vi "ArduinoLT_Collect_Control.vi"(7 "Arduino Configuration":T2={"Lights: Digital I/O Pins"={"Coaxial"=0, "Spotlights"=0}, "Thermistor Settings"={"Analogue Readout Pin"=1, "Vcc Reference Pin"=0, "Paired Resistance (10K Ohms)"=10000.0, "Units (C)"=enum."Celsius"}} {"Thermistor Settings"."Paired Resistance (10K Ohms)" format="%#_13g"}, 8 "error in":errorcluster, 9 "Arduino Resource IN":T3={"VISA resource"="", "Board Type"=enum."Uno", "Connection Type"=enum."USB / Serial", "Bytes Per Packet (15)"=15}, 10 "Spotlights":bool, 11 "Coaxial light":bool) -> (0 "error out":errorcluster, 1 "Arduino Resource OUT":T3={"VISA resource"="COM11", "Board Type"=enum."Uno", "Connection Type"=enum."USB / Serial", "Bytes Per Packet (15)"=15}, 3 "Thermometer [C]":dbl(slide) scale=0.0..50.0)   [LabVIEW 2016]
uses:
  <vilib>/LabVIEW Interface for Arduino/Type Defs/Arduino Resource.ctl
  <vilib>/LabVIEW Interface for Arduino/Type Defs/Board Type.ctl
  Controls/ArduinoLT-ConfigurationControl.ctl
  <vilib>/LabVIEW Interface for Arduino/LabVIEW Interface for Arduino.lvlib
panel:
  in  "Tab Control":T1(tab)
  out "VCC [V]":dbl=5.0 format="%#_13g"
  # "LIGHTS"
  # "TEMPERATURE"
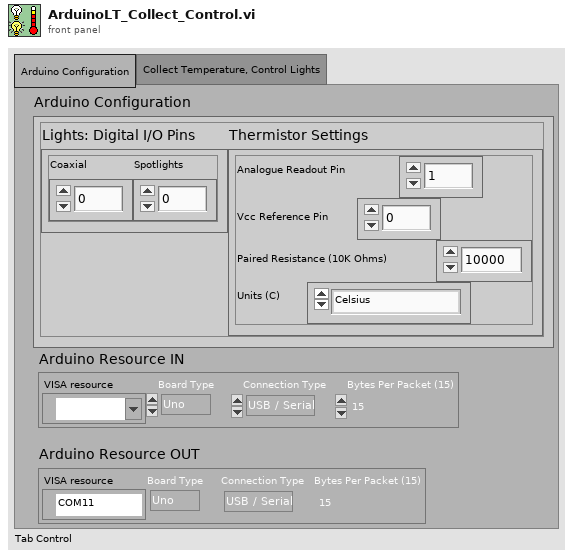
[diagram p1: front panel]
types:
  T1 = enum32{"Arduino Configuration", "Collect Temperature, Control Lights"}
  T2 = typedef "ArduinoLT-ConfigurationControl.ctl" = cluster{"Lights: Digital I/O Pins":cluster{"Coaxial":u8, "Spotlights":u8}, "Thermistor Settings":cluster{"Analogue Readout Pin":u8, "Vcc Reference Pin":u8, "Paired Resistance (10K Ohms)":dbl, "Units (C)":enum16{"Celsius", "Fahrenheit", "Kelvin"}}}
  T3 = typedef "LabVIEW Interface for Arduino.lvlib/Arduino Resource.ctl" = cluster{"VISA resource":refnum<visa-resource-name>, "Board Type":T4, "Connection Type":enum8{"USB / Serial"}, "Bytes Per Packet (15)":u8}
  T4 = typedef "LabVIEW Interface for Arduino.lvlib/Board Type.ctl" = enum16{"Uno", "Dimuelanove w/Atmega 328", "Mega 2560"}
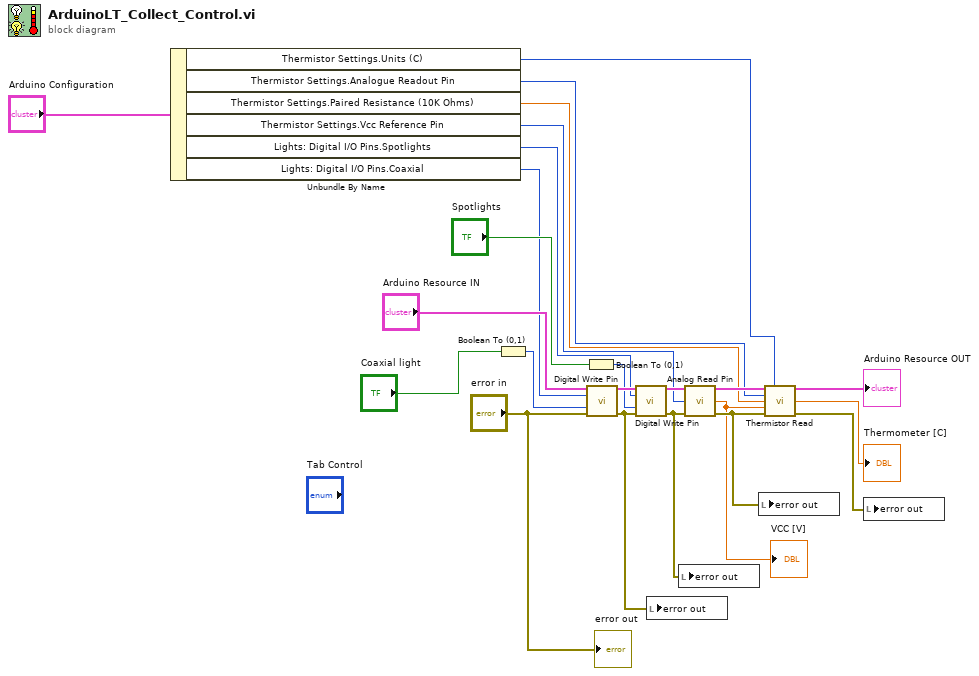
[diagram p0: block diagram]
diagram:
  n1 = Unbundle By Name("Arduino Configuration") -> ("Thermistor Settings.Units (C)"=w3:enum16{"Celsius", "Fahrenheit", "Kelvin"}, "Thermistor Settings.Analogue Readout Pin"=w4:u8, "Thermistor Settings.Paired Resistance (10K Ohms)"=w5:dbl, "Thermistor Settings.Vcc Reference Pin"=w6:u8, "Lights: Digital I/O Pins.Spotlights"=w7:u8, "Lights: Digital I/O Pins.Coaxial"=w8:u8)
  n2 = Boolean To (0,1)(Boolean="Coaxial light") -> (0, 1=w18:i16)
  n3 = Boolean To (0,1)(Boolean="Spotlights") -> (0, 1=w17:i16)
  n4 = call <vilib>:"Digital Write Pin.vi"("Arduino Resource"="Arduino Resource IN", "Digital I/O Pin (0)"=w8, "Value (0)"=w18, "error in"="error in") -> ("Arduino Resource"=w20:T3, "error out"=w11:errorcluster)  [unwired: 10 in]
  n5 = call <vilib>:"Digital Write Pin.vi"("Arduino Resource"=w20, "Digital I/O Pin (0)"=w7, "Value (0)"=w17, "error in"=w11) -> ("Arduino Resource"=w16:T3, "error out"=w12:errorcluster)  [unwired: 10 in]
  n6 = local write "error out"(w11) -> ()
  n7 = local write "error out"(w12) -> ()
  n8 = call <vilib>:"Analog Read Pin.vi"("Arduino Resource"=w16, "Analog Input Pin (0)"=w6, "error in"=w12) -> ("Arduino Resource"=w15:T3, "Voltage"=w1:dbl, "error out"=w13:errorcluster)  [unwired: 10 in]
  "VCC [V]" <- w1
  n9 = local write "error out"(w13) -> ()
  n10 = call <vilib>:"Thermistor Read.vi"("Arduino Resource"=w15, "Units (C)"=w3, "Thermistor AI Pin (0)"=w4, "Paired Resistance (10K Ohms)"=w5, "Vcc (5 v)"=w1, "error in"=w13) -> ("Arduino Resource"=→"Arduino Resource OUT":T3, "Temperature"=→"Thermometer [C]":dbl, "error out"=w22:errorcluster)  [unwired: 7 in]
  n11 = local write "error out"(w22) -> ()
  "error out" <- "error in"
